vi "Create_Pfeiffer_Save_Files.vi"(8 "error in (no error)":errorcluster, 11 "base path":path) -> (0 "error out":errorcluster, 1 "New Folder Created?":bool, 2 "Ref Num Array":refnum<file>[](array[refnum]), 3 "Save Files Array":path[](array[path]), 4 "Scan Number":i32)   [LabVIEW 2015]
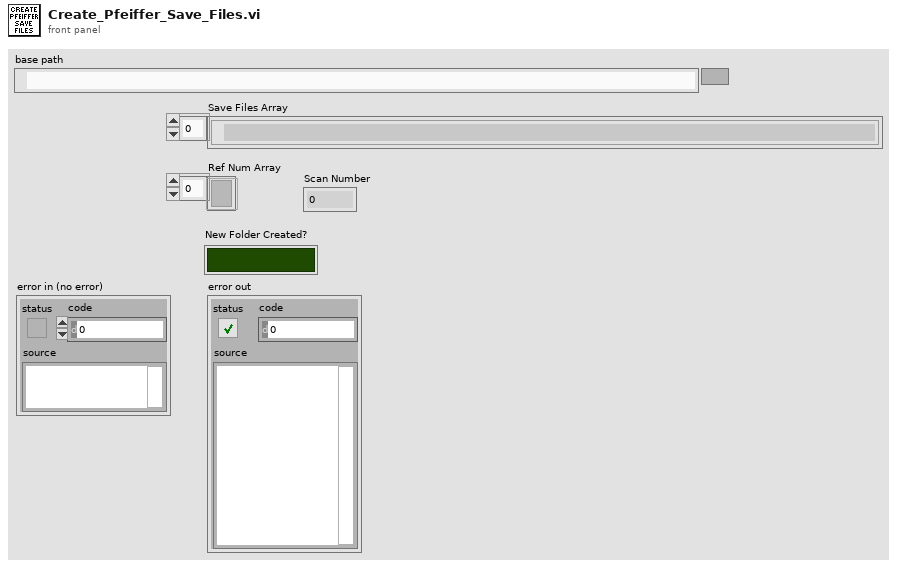
[diagram p1: front panel]
types:
  T1 = enum16{"open", "replace", "create", "open or create", "replace or create", "replace or create with confirmation"}
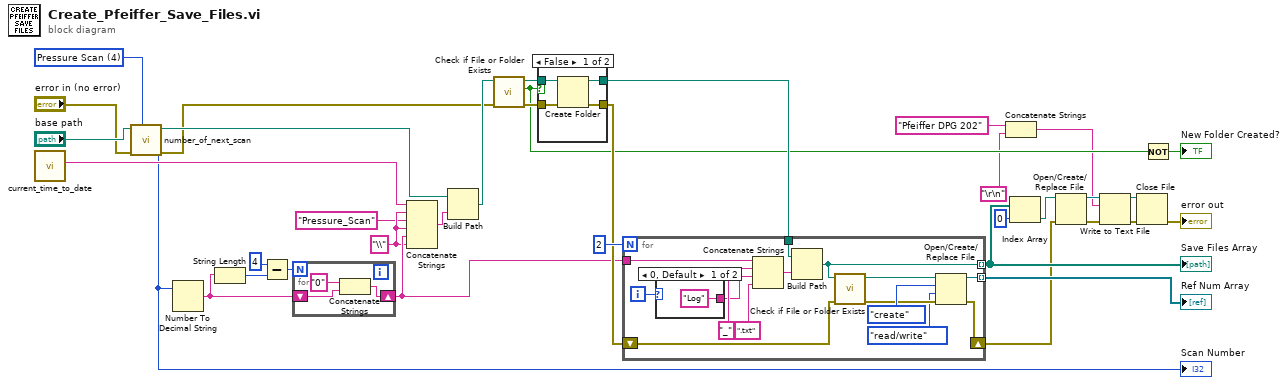
[diagram p0: block diagram]
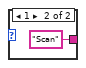
[diagram p3: hidden frame]
diagram:
  w2 = u16 4 items=["Energy / Time", "Motor", "TDC", "Keithley", "Pressure Scan"] ("Scan Type")
  w22 = "\\" ("string")
  n1 = call "current_time_to_date.vi"() -> ("yyyy-mm-dd"=w31:string)  [unwired: 10 in, 1 out]
  n2 = call "number_of_next_scan.vi"("Scan Type"=w2, "error in (no error)"="error in (no error)", "base path"="base path") -> ("error out"=w16:errorcluster, "scan nr"=w5:i32, "path out"=w18:path)  [unwired: 6 in]
  "Scan Number" <- w5
  n3 = Number To Decimal String(number=w5) -> (decimal integer string=w33:string)  [unwired: 1 in]
  n4 = String Length(string=w33) -> (length=w36:i32)
  n5 = Subtract(x=4, y=w36) -> (x-y=w34:i32)
  n6 = for {
    N: w34 -> [_]
    shift-right: [w37] -> w23
    shift-left: w33 -> [w38]
    n7 = Concatenate Strings("0", w38) -> (w37:string)
  }
  n8 = Concatenate Strings(w31, w22, "Pressure_Scan" ("string"), w22, w23, w22) -> (w26:string)
  n9 = Build Path(base path=w18, name or relative path=w26) -> (appended path=w30:path)
  n10 = call <vilib>:"Check if File or Folder Exists.vi"("error in (no error)"=w16, "path"=w30) -> ("error out"=w27:errorcluster, "file or folder exists?"=w21:bool, "dup path"=w29:path)  [unwired: 7 in]
  n11 = case shown="False" w21 {
    tunnel: w29 -> [w43 w45]
    tunnel: [w42 w45] -> w28
    tunnel: w27 -> [w41 w44]
    tunnel: [w40 w44] -> w25
    frame False {
      n12 = Create Folder(path (use dialog)=w43, error in=w41) -> (created path=w42:path, error out=w40:errorcluster)  [unwired: 1 in, 1 out]
    }
    frame True {
    }
  }
  n13 = for {
    N: 2 -> [_]
    tunnel: w23 -> [w59]
    tunnel: w28 -> [w58]
    tunnel: [w53] -> w15 mode=indexing
    shift-right: [w48] -> w8
    shift-left: w25 -> [w49]
    tunnel: [w46] -> w24 mode=indexing
    i -> [w55]
    n14 = case shown="0, Default" w55 {
      tunnel: ["Log" ("string") "Scan" ("string")] -> w54
      frame 0, Default {
      }
      frame 1 {
      }
    }
    n15 = Concatenate Strings(w59, "_" ("string"), w54, ".txt" ("string")) -> (w60:string)
    n16 = Build Path(base path=w58, name or relative path=w60) -> (appended path=w53:path)
    n17 = call <vilib>:"Check if File or Folder Exists.vi"("error in (no error)"=w49, "path"=w53) -> ("error out"=w50:errorcluster, "dup path"=w52:path)  [unwired: 7 in, 1 out]
    n18 = Open/Create/Replace File(file path (use dialog)=w52, error in=w50, operation (0:open)=T1."create", access (0:read/write)=enum16{"read/write", "read-only", "write-only"}."read/write") -> (refnum out=w46:refnum<file>, error out=w48:errorcluster)  [unwired: 2 in, 1 out]
  }
  "Save Files Array" <- w15
  "Ref Num Array" <- w24
  n19 = Concatenate Strings("Pfeiffer DPG 202" ("string"), "\r\n") -> (w6:string)
  n20 = Index Array(array=w15, index=0) -> (element=w13:path)
  n21 = Open/Create/Replace File(file path (use dialog)=w13, error in=w8) -> (refnum out=w11:refnum<file>, error out=w12:errorcluster)  [unwired: 4 in, 1 out]
  n22 = Write to Text File(file (use dialog)=w11, text=w6, error in=w12) -> (refnum out=w10:refnum<file>, error out=w9:errorcluster)  [unwired: 1 in, 1 out]
  n23 = Close File(refnum=w10, error in=w9) -> (error out=→"error out":errorcluster)  [unwired: 1 out]
  n24 = Not(x=w21) -> (.not. x?=→"New Folder Created?":bool)
